vi "SubVI Find Slave and Channel.vi"(10 "NewVal":bool[][](array[boolean]), 11 "OldVal":bool[][](array[boolean])) -> (1 "Value ON/OFF":bool, 2 "Slave":i32, 3 "Channel":i16)   [LabVIEW 2020, in "QuPMXdriver.lvlib"]
doc: "Finds which array element changed, returns the element and slave and channel index.\n(Channels are rows, slaves are collumns)"
uses:
  QuPMXdriver.lvlib
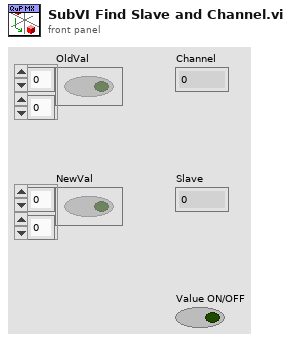
[diagram p1: front panel]
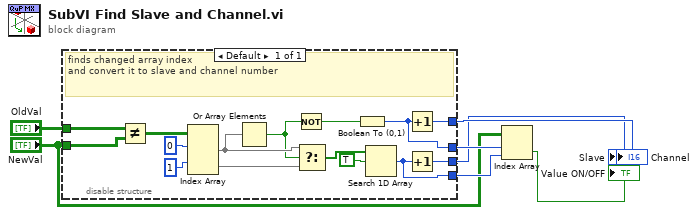
[diagram p0: block diagram]
diagram:
  n1 = disable-structure shown="Default" {
    disable-tunnel: "OldVal" -> [w22]
    disable-tunnel: "NewVal" -> [w21]
    disable-tunnel: [w11] -> w2
    disable-tunnel: [w10] -> w3
    disable-tunnel: [w9] -> w7
    disable-tunnel: [w8] -> w6
    frame Enabled {
      # "finds changed array index\nand convert it to slave and channel number"
      n2 = Not Equal?(x=w22, y=w21) -> (x != y?=w20:bool[][])
      n3 = Index Array(array=w20, index (row) #1=0 ("index (row)"), index (row) #2=1 ("index (row)")) -> (element #1=w17:bool[], element #2=w16:bool[])  [unwired: 2 in]
      n4 = Or Array Elements(Boolean array=w17) -> (logical OR=w13:bool)
      n5 = Not(x=w13) -> (.not. x?=w12:bool)
      n6 = Select(t=w17, s=w13, f=w16) -> (s? t:f=w15:bool[])
      n7 = Boolean To (0,1)(Boolean=w12) -> (0, 1=w8:i16)
      n8 = Search 1D Array(1D array=w15, element=TRUE) -> (index of element=w9:i32)  [unwired: 1 in]
      n9 = Increment(x=w8) -> (x+1=w10:i16)
      n10 = Increment(x=w9) -> (x+1=w11:i32)
    }
  }
  "Channel" <- w3
  "Slave" <- w2
  n11 = Index Array(array="NewVal", index (row)=w6, index (col)=w7) -> (element=→"Value ON/OFF":bool)
